vi "LOC subReadWriteVIStringINIKeys(Path).vi"(4 "Mode":enum16{"Read", "Write"}(ring), 5 "Section":string, 6 "error in (no error)":errorcluster, 8 "ConfigFileRefnum":T1, 9 "ControlRefnum":refnum<vi>) -> (0 "error out":errorcluster)   [LabVIEW 2020, in "Localization_Tools.lvlib"]
uses:
  Localization_Tools.lvlib
  <vilib>/Utility/config.llb/Config Data RefNum.ctl
  <vilib>/Utility/config.llb/NI_LVConfig.lvlib
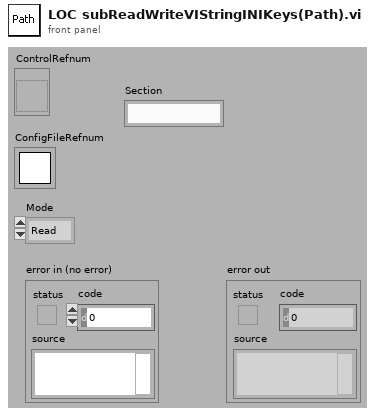
[diagram p1: front panel]
types:
  T1 = typedef "NI_LVConfig.lvlib/Config Data RefNum.ctl" = refnum<k1>
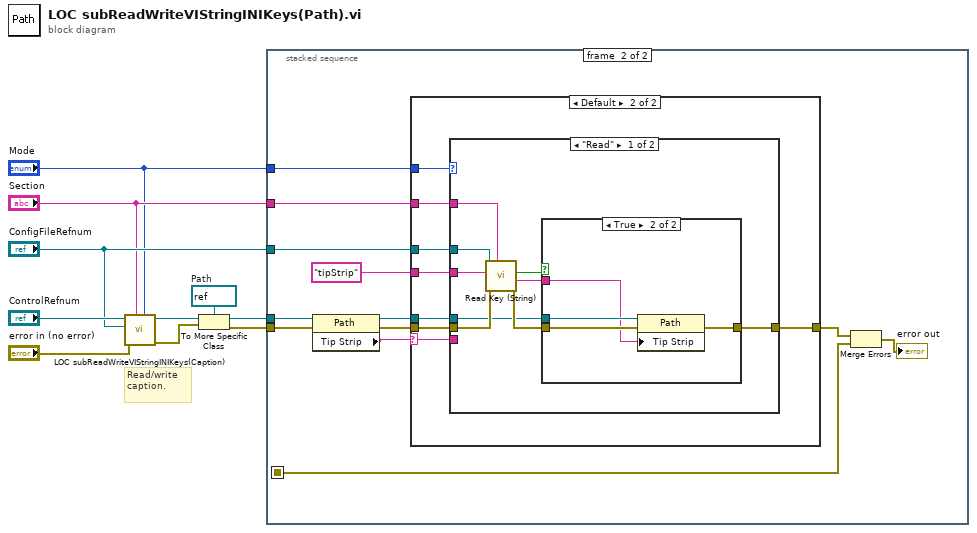
[diagram p0: block diagram]
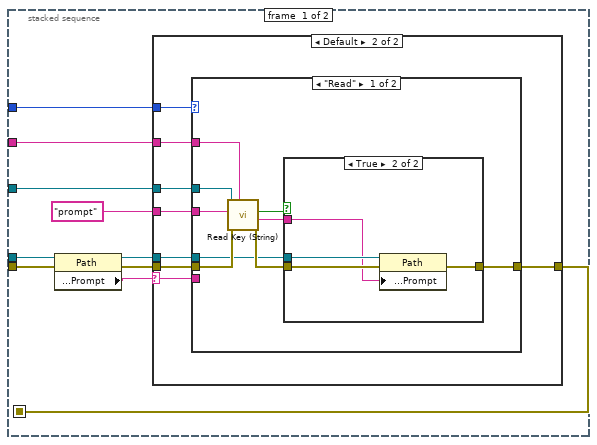
[diagram p2: hidden frame]
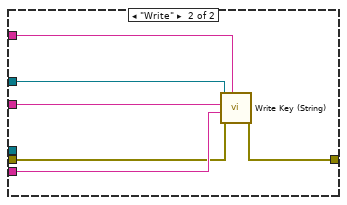
[diagram p5: hidden frame]
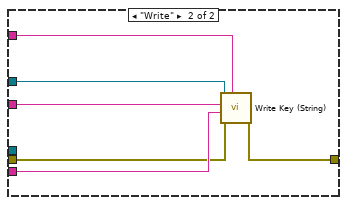
[diagram p8: hidden frame]
diagram:
  w5 = refnum<vi> refnum  # Path
  # "Read/write\ncaption."
  n1 = call "LOC subReadWriteVIStringINIKeys(Caption).vi"("Mode"="Mode", "Section"="Section", "error in (no error)"="error in (no error)", "ConfigFileRefnum"="ConfigFileRefnum", "ControlRefnum"="ControlRefnum") -> ("error out"=w3:errorcluster, "dup ControlRefnum"=w4:refnum<vi>)  [unwired: 3 in]
  n2 = To More Specific Class(target class=w5, reference=w4, error in=w3) -> (specific class reference=w2:refnum<vi>, error out=w1:errorcluster)
  n3 = stacked-sequence {
    seq-local: [w11 _] -> [_ w51]
    tunnel: "ConfigFileRefnum" -> [w20 w61]
    tunnel: "Section" -> [w19 w60]
    tunnel: "Mode" -> [w18 w59]
    tunnel: w2 -> [w17 w58]
    tunnel: w1 -> [w16 w57]
    frame #0 {
      n4 = property class="Path"(reference=w17, error in=w16) -> (reference out=w12:refnum<vi>, error out=w13:errorcluster, "Browse Options:Prompt"=w15:string)
      n5 = case shown="Default" w15 {
        selector: w15 -> [_ w24]
        tunnel: "prompt" ("key") -> [_ w29]
        tunnel: w20 -> [_ w28]
        tunnel: w19 -> [_ w27]
        tunnel: w18 -> [_ w26]
        tunnel: [w21 w25] -> w11
        tunnel: w13 -> [w21 w23]
        tunnel: w12 -> [_ w22]
        frame "" {
          # "no prompt, don't need to read/write\nthe ini entry."
        }
        frame Default {
          n6 = case shown="\"Read\"" w26 {
            tunnel: w28 -> [w38 w49]
            tunnel: w27 -> [w37 w47]
            tunnel: w29 -> [w36 w48]
            tunnel: [w34 w46] -> w25
            tunnel: w23 -> [w32 w44]
            tunnel: w24 -> [_ w45]
            tunnel: w22 -> [w30 _]
            frame "Read" {
              n7 = call <vilib>:"Read Key (String).vi"("section"=w37, "error in (no error)"=w32, "key"=w36, "refnum"=w38) -> ("error out"=w35:errorcluster, "value"=w33:string, "found?"=w31:bool)  [unwired: 4 in, 1 out]
              n8 = case shown="True" w31 {
                tunnel: w35 -> [w39 w43]
                tunnel: [w39 w42] -> w34
                tunnel: w33 -> [_ w40]
                tunnel: w30 -> [_ w41]
                frame False {
                }
                frame True {
                  n9 = property class="Path"(reference=w41, error in=w43, "Browse Options:Prompt"=w40) -> (error out=w42:errorcluster)  [unwired: 1 out]
                }
              }
            }
            frame "Write" {
              n10 = call <vilib>:"Write Key (String).vi"("section"=w47, "error in (no error)"=w44, "value"=w45, "key"=w48, "refnum"=w49) -> ("error out"=w46:errorcluster)  [unwired: 4 in, 2 out]
            }
          }
        }
      }
    }
    frame #1 {
      n11 = property class="Path"(reference=w58, error in=w57) -> (reference out=w53:refnum<vi>, error out=w54:errorcluster, "Tip Strip"=w56:string)
      n12 = case shown="Default" w56 {
        selector: w56 -> [_ w65]
        tunnel: "tipStrip" ("key") -> [_ w70]
        tunnel: w61 -> [_ w69]
        tunnel: w60 -> [_ w68]
        tunnel: w59 -> [_ w67]
        tunnel: [w62 w66] -> w52
        tunnel: w54 -> [w62 w64]
        tunnel: w53 -> [_ w63]
        frame "" {
          # "no tipstrip, don't need to read/write\nthe ini entry."
        }
        frame Default {
          n13 = case shown="\"Read\"" w67 {
            tunnel: w69 -> [w79 w90]
            tunnel: w68 -> [w78 w88]
            tunnel: w70 -> [w77 w89]
            tunnel: [w75 w87] -> w66
            tunnel: w64 -> [w73 w85]
            tunnel: w65 -> [_ w86]
            tunnel: w63 -> [w71 _]
            frame "Read" {
              n14 = call <vilib>:"Read Key (String).vi"("section"=w78, "error in (no error)"=w73, "key"=w77, "refnum"=w79) -> ("error out"=w76:errorcluster, "value"=w74:string, "found?"=w72:bool)  [unwired: 4 in, 1 out]
              n15 = case shown="True" w72 {
                tunnel: w76 -> [w80 w84]
                tunnel: [w80 w83] -> w75
                tunnel: w74 -> [_ w81]
                tunnel: w71 -> [_ w82]
                frame False {
                }
                frame True {
                  n16 = property class="Path"(reference=w82, error in=w84, "Tip Strip"=w81) -> (error out=w83:errorcluster)  [unwired: 1 out]
                }
              }
            }
            frame "Write" {
              n17 = call <vilib>:"Write Key (String).vi"("section"=w88, "error in (no error)"=w85, "value"=w86, "key"=w89, "refnum"=w90) -> ("error out"=w87:errorcluster)  [unwired: 4 in, 2 out]
            }
          }
        }
      }
      n18 = Merge Errors(w52, w51) -> (→"error out":errorcluster)
    }
  }
